vi "PostUninstall.vi"(10 "Variant":variant) -> (0 "error out":errorcluster)   [LabVIEW 2012]
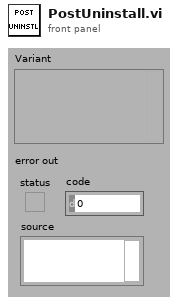
[diagram p1: front panel]
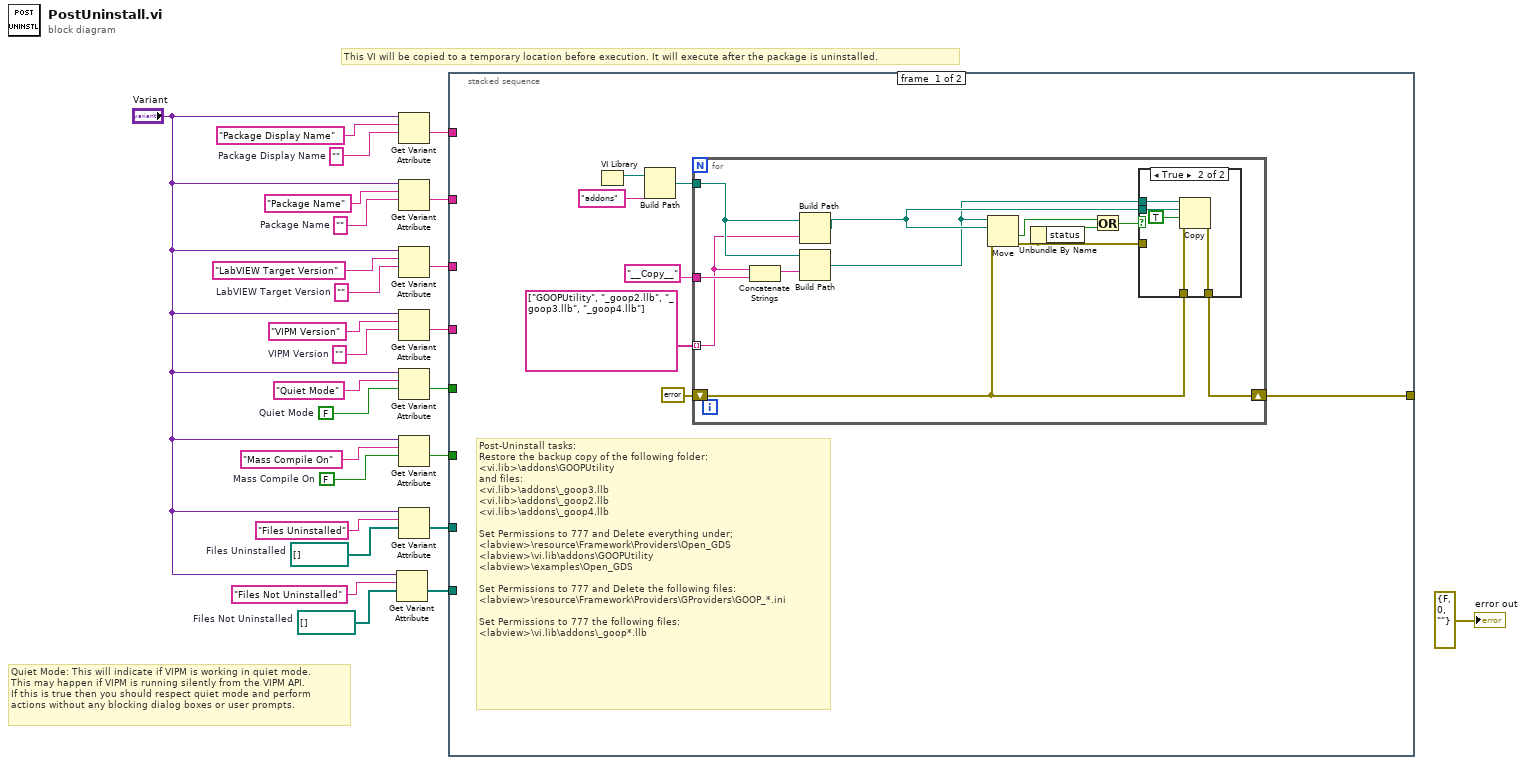
[diagram p0: block diagram]
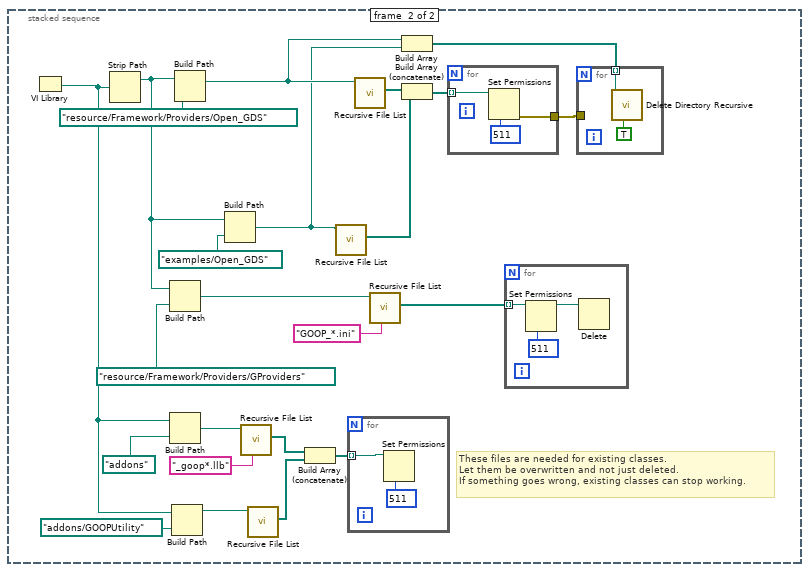
[diagram p3: hidden frame]
diagram:
  w1 = path[] []  # Files Not Uninstalled
  w2 = path[] []  # Files Uninstalled
  w8 = FALSE  # Mass Compile On
  w9 = ""  # Package Display Name
  w16 = FALSE  # Quiet Mode
  w19 = ""  # VIPM Version
  w21 = ""  # LabVIEW Target Version
  w23 = ""  # Package Name
  # "Quiet Mode: This will indicate if VIPM is working in quiet mode.\nThis may happen if VIPM is running silently from the VIPM API.\nIf this is true then you should respect quiet mode and perform\nactions without any blocking dialog boxes or user prompts."
  # "This VI will be copied to a temporary location before execution. It will execute after the package is uninstalled."
  n1 = Get Variant Attribute(Variant="Variant", name="Files Not Uninstalled", default value (empty Variant)=w1) -> (value=w6:path[])  [unwired: 1 in, 3 out]
  n2 = Get Variant Attribute(Variant="Variant", name="Package Display Name", default value (empty Variant)=w9) -> (value=w15:string)  [unwired: 1 in, 3 out]
  n3 = Get Variant Attribute(Variant="Variant", name="Package Name", default value (empty Variant)=w23) -> (value=w14:string)  [unwired: 1 in, 3 out]
  n4 = Get Variant Attribute(Variant="Variant", name="LabVIEW Target Version", default value (empty Variant)=w21) -> (value=w13:string)  [unwired: 1 in, 3 out]
  n5 = Get Variant Attribute(Variant="Variant", name="VIPM Version", default value (empty Variant)=w19) -> (value=w12:string)  [unwired: 1 in, 3 out]
  n6 = Get Variant Attribute(Variant="Variant", name="Quiet Mode", default value (empty Variant)=w16) -> (value=w11:bool)  [unwired: 1 in, 3 out]
  n7 = Get Variant Attribute(Variant="Variant", name="Mass Compile On", default value (empty Variant)=w8) -> (value=w10:bool)  [unwired: 1 in, 3 out]
  n8 = Get Variant Attribute(Variant="Variant", name="Files Uninstalled", default value (empty Variant)=w2) -> (value=w5:path[])  [unwired: 1 in, 3 out]
  n9 = stacked-sequence {
    tunnel: w15 -> [_ _]
    tunnel: w14 -> [_ _]
    tunnel: w13 -> [_ _]
    tunnel: w12 -> [_ _]
    tunnel: w11 -> [_ _]
    tunnel: w10 -> [_ _]
    tunnel: w5 -> [_ _]
    tunnel: w6 -> [_ _]
    tunnel: [w27 _] -> _
    frame #0 {
      # "Post-Uninstall tasks:\nRestore the backup copy of the following folder:\n<vi.lib>\\addons\\GOOPUtility\nand files:\n<vi.lib>\\addons\\_goop3.llb\n<vi.lib>\\addons\\_goop2.llb\n<vi.lib>\\addons\\_goop4.llb\n\nSet Permissions to 777 and Delete everything under;\n<labview>\\resource\\Framework\\Providers\\Open_GDS\n<labview>\\vi.lib\\addons\\GOOPUtility\n<labview>\\examples\\Open_GDS\n\nSet Permissions to 777 and Delete the following files:\n<labview>\\resource\\Framework\\Providers\\GProviders\\GOOP_*.ini\n\nSet Permissions to 777 the following files:\n<labview>\\vi.lib\\addons\\_goop*.llb"
      n10 = VI Library() -> (path=w29:path)
      n11 = Build Path(base path=w29, name or relative path="addons") -> (appended path=w32:path)
      n12 = for {
        tunnel: "__Copy__" ("name or relative path") -> [w41]
        tunnel: w32 -> [w39]
        tunnel: string[] ["GOOPUtility", "_goop2.llb", "_goop3.llb", "_goop4.llb"] -> [w38] mode=indexing
        shift-right: [w36] -> w27
        shift-left: errorcluster {"status"=FALSE, "code"=0, "source"=""} ("error out") -> [w37]
        n13 = Concatenate Strings(w38, w41) -> (w40:string)
        n14 = Build Path(base path=w39, name or relative path=w38) -> (appended path=w35:path)
        n15 = Build Path(base path=w39, name or relative path=w40) -> (appended path=w34:path)
        n16 = Move(source path=w34, error in=w37, 10:w35) -> (error out=w42:errorcluster, 1:w44:bool)  [unwired: 2 in, 1 out]
        n17 = Unbundle By Name(w42) -> ("status"=w45:bool)
        n18 = Or(x=w44, y=w45) -> (x .or. y?=w43:bool)
        n19 = case shown="True" w43 {
          tunnel: w42 -> [w46 _]
          tunnel: [w46 w50] -> w36
          tunnel: w37 -> [_ w49]
          tunnel: w34 -> [_ w48]
          tunnel: w35 -> [_ w47]
          frame False {
          }
          frame True {
            n20 = Copy(8:w49, 9:TRUE ("overwrite (F)"), 10:w47, 11:w48) -> (0:w50:errorcluster)  [unwired: 1 in, 2 out]
          }
        }
      }
    }
    frame #1 {
      # "These files are needed for existing classes.\nLet them be overwritten and not just deleted.\nIf something goes wrong, existing classes can stop working."
      n21 = VI Library() -> (path=w57:path)
      n22 = Strip Path(path=w57) -> (stripped path=w65:path)  [unwired: 1 out]
      n23 = Build Path(base path=w65, name or relative path=path "resource/Framework/Providers/GProviders" ("path")) -> (appended path=w62:path)
      n24 = Build Path(base path=w57, name or relative path=path "addons" ("path")) -> (appended path=w58:path)
      n25 = Build Path(base path=w57, name or relative path=path "addons/GOOPUtility" ("path")) -> (appended path=w52:path)
      n26 = Build Path(base path=w65, name or relative path=path "resource/Framework/Providers/Open_GDS" ("path")) -> (appended path=w71:path)
      n27 = Build Path(base path=w65, name or relative path=path "examples/Open_GDS" ("path")) -> (appended path=w64:path)
      n28 = call <vilib>:"Recursive File List.vi"("pattern"="_goop*.llb", "Folder Path"=w58) -> ("All Files in Dir"=w54:path[])  [unwired: 5 in, 4 out]
      n29 = call <vilib>:"Recursive File List.vi"("Folder Path"=w52) -> ("All Files in Dir"=w55:path[])  [unwired: 6 in, 4 out]
      n30 = Build Array (concatenate)(w54, w55) -> (w53:path[])
      n31 = call <vilib>:"Recursive File List.vi"("Folder Path"=w64) -> ("All Files in Dir"=w63:path[])  [unwired: 6 in, 4 out]
      n32 = for {
        tunnel: w53 -> [w75] mode=indexing
        n33 = Set Permissions(7:i16 511 ("permissions"), 11:w75) -> ()  [unwired: 3 in, 2 out]
      }
      n34 = call <vilib>:"Recursive File List.vi"("Folder Path"=w71) -> ("All Files in Dir"=w73:path[])  [unwired: 6 in, 4 out]
      n35 = call <vilib>:"Recursive File List.vi"("pattern"="GOOP_*.ini", "Folder Path"=w62) -> ("All Files in Dir"=w60:path[])  [unwired: 5 in, 4 out]
      n36 = Build Array(w71, w64) -> (w69:path[])
      n37 = Build Array (concatenate)(w73, w63) -> (w72:path[])
      n38 = for {
        tunnel: w72 -> [w81] mode=indexing
        tunnel: [w79] -> w70
        n39 = Set Permissions(7:i16 511 ("permissions"), 11:w81) -> (0:w79:errorcluster)  [unwired: 3 in, 1 out]
      }
      n40 = for {
        tunnel: w60 -> [w82] mode=indexing
        n41 = Set Permissions(7:i16 511 ("permissions"), 11:w82) -> (3:w84:path)  [unwired: 3 in, 1 out]
        n42 = Delete(path (use dialog)=w84) -> ()  [unwired: 4 in, 3 out]
      }
      n43 = for {
        tunnel: w70 -> [_]
        tunnel: w69 -> [w78] mode=indexing
        n44 = call <vilib>:"Delete Directory Recursive.vi"("keep deleting on error? (F)"=TRUE, "Folder to Delete"=w78) -> ()  [unwired: 8 in, 2 out]
      }
    }
  }
  "error out" <- errorcluster {"status"=FALSE, "code"=0, "source"=""} ("error out")
